vi "SMO.InstrumentDriver VI Tree.vi"   [LabVIEW 2013, in "SMO.InstrumentDriver.lvclass"]
uses:
  SMO.InstrumentDriver.lvclass
  Typedefs/WriteData.ctl
panel:
  # "SEE DIAGRAM\nFOR VI Tree"
types:
  T1 = typedef "SMO.InstrumentDriver.lvclass/WriteData.ctl" = dbl
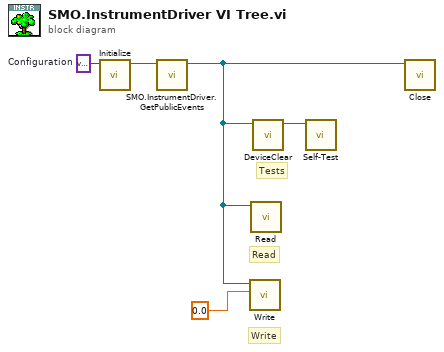
[diagram p0: block diagram]
diagram:
  w3 = variant  # Configuration
  # "Write"
  # "Tests"
  # "Read"
  n1 = call "Initialize.vi"("Configuration"=w3) -> ("SMO.InstrumentDriver out"=w5:refnum<class "SMO.InstrumentDriver.lvclass">)  [unwired: 8 in, 2 out]
  n2 = call "SMO.InstrumentDriver.GetPublicEvents.vi"("SMO.Instrument"=w5) -> ("SMO.Instrument out"=w2:refnum<class "SMO.InstrumentDriver.lvclass">)  [unwired: 8 in, 2 out]
  n3 = call "Write.vi"("Write"=T1 0.0, "SMO.InstrumentDriver"=w2) -> ()  [unwired: 8 in, 2 out]
  n4 = call "Read.vi"("SMO.Instrument"=w2) -> ()  [unwired: 8 in, 3 out]
  n5 = call "DeviceClear.vi"("SMO.Instrument"=w2) -> ("SMO.Instrument out"=w4:refnum<class "SMO.InstrumentDriver.lvclass">)  [unwired: 9 in, 1 out]
  n6 = call "Self-Test.vi"("SMO.Instrument"=w4) -> ()  [unwired: 9 in, 2 out]
  n7 = call "Close.vi"("SMO.InstrumentDriver in"=w2) -> ()  [unwired: 10 in, 1 out]
